vi "Open Image Sequence Test Bench.vi"   [LabVIEW 2017]
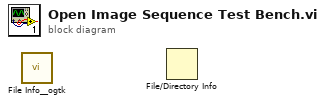
[diagram p0: block diagram]
diagram:
  n1 = call <userlib>:"File Info__ogtk.vi"() -> ()  [unwired: 6 in, 3 out]
  n2 = File/Directory Info() -> ()  [unwired: 2 in, 7 out]
